vi "write tag by index.vi"(8 "error in":errorcluster, 9 "tag":refnum<class "tag descriptor.lvclass">, 10 "index":i32, 11 "tag collection in":refnum<class "tag collection.lvclass">) -> (0 "error out":errorcluster, 3 "tag collection out":refnum<class "tag collection.lvclass">)   [LabVIEW 2013, in "tag bus.lvlib" / "tag collection.lvclass"]
uses:
  tag collection.lvclass
  tag/tag descriptor.lvclass
  tag collection.lvclass/tag collection.ctl
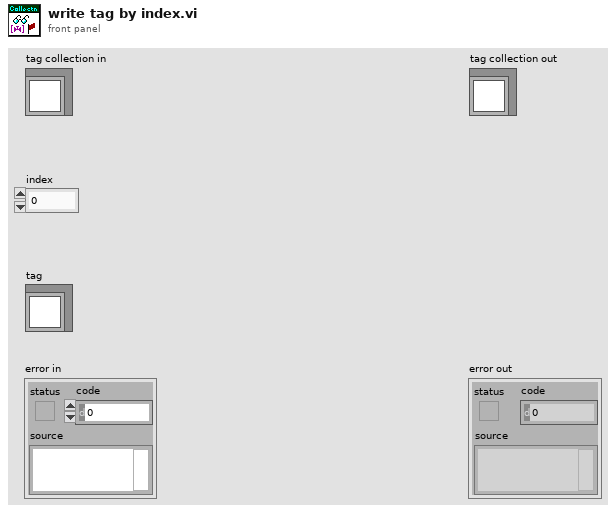
[diagram p1: front panel]
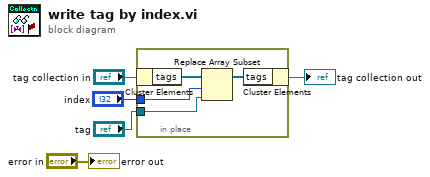
[diagram p0: block diagram]
diagram:
  n1 = in-place {
    in-place-border: "index" -> [w7]
    in-place-border: "tag" -> [w6]
    n2 = in-place-cluster #1("tag collection in") -> ("tags"=w9:refnum<class "tag descriptor.lvclass">[])
    n3 = Replace Array Subset(array=w9, new element=w6, index=w7) -> (w8:refnum<class "tag descriptor.lvclass">[])
    n4 = in-place-cluster #1("tags"=w8) -> (→"tag collection out":refnum<class "tag collection.lvclass">)
  }
  "error out" <- "error in"
